vi "PH_Beckhoff.destructor.vi"(0 "i ref in":refnum<vi>, 5 "error in(no error)":errorcluster) -> (19 "error out":errorcluster)   [LabVIEW 2014, in "PH_Beckhoff.lvlib"]
doc: "This is the destructor of a class.\n\nLicense Agreement for this software:\n\nCopyright (C)\nGesellschaft für Schwerionenforschung, GSI\nPlanckstr. 1\n64291 Darmstadt\nGermany\n\nContact: D.Beck@gsi.de \n\nThis program is free software; you can redistribute it and/or modify it under the terms of the \nGNU General Public License as published by the Free Software Foundation; either version 2 of \nthe license, or (at your option) any later version.\n\nThis program is distributed in the hope that it will be useful, but WITHOUT ANY WARRANTY; \nwithout even the implied warranty of MERCHANTABILITY or FITNESS FOR A PARTICULAR PURPOSE. See the GNU General License for more details (http://www.gnu.org).\n\nGesellschaft für Schwerionenforschung, GSI\nPlanckstr. 1, 64291 Darmstadt, Germany\nFor all questions and ideas contact: M.Richter@gsi.de, H.Brand@gsi.de or D.Beck@gsi.de.\nLast update: 16-JUN-2004"
uses:
  PH_Beckhoff.lvlib
  non_GPL/instr.lib/Beckhoff/Beckhoff - Driver np.lvlib
  lib.lib/DimLVEvent/LVDimInterface/LVDimInterface.lvlib
  PH_Class/PH_Class.lvlib
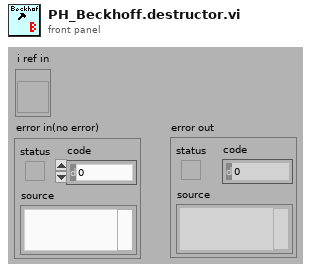
[diagram p1: front panel]
types:
  T1 = typedef "PH_Beckhoff.lvlib/PH_Beckhoff.i attribute.ctl" = cluster{"GUI Refs":T2, "operation?":bool, "Default Prdc Interval":i32, "Connection":T3, "AMS Net ID":T4, "Klemmencluster: # of":T5, "Values":T6, "IP":string, "Description":string, "configured?":bool, "Change Manager":cluster{"Detemination wanted?":bool, "Values changed at":cluster{"Sonderklemmen Inputs":i32[], "Analog Inputs":i32[], "Analog Outputs":i32[], "Digital Inputs":i32[], "Digital Outputs":i32[]}}, "Difference to handle an analog input as change":u32}
  T2 = typedef "PH_Beckhoff.lvlib/PH_Beckhoff.GUI Refs.ctl" = cluster{"ADS Error":refnum<vi>, "Values":refnum<vi>, "configured?":refnum<vi>, "Connection":refnum<vi>, "IP":refnum<vi>, "Prdc Int [ms]":refnum<vi>}
  T3 = typedef "PH_Beckhoff.lvlib/PH_Beckhoff.Connectivity.ctl" = cluster{"DLL?":bool, "Port?":bool, "Client?":bool, "Ping?":bool, "unsuccessful Pings":u32}
  T4 = typedef "Beckhoff - Driver np.lvlib/Beckhoff Access.ctl" = cluster{"DLL path":path, "AMS Net ID":cluster{"1st # of IP":u8, "2nd # of IP":u8, "3rd # of IP":u8, "4th # of IP":u8, "In Port":u8, "Out Port":u8}}
  T5 = typedef "Beckhoff - Driver np.lvlib/Klemmendeclarer.ctl" = cluster{"Offset due to Sonderklemms":u32, "analog Inputs":u32, "analog Outputs":u32, "digital Input Bits":u32, "digital Output Bits":u32}
  T6 = typedef "PH_Beckhoff.lvlib/PH_Beckhoff.Values.ctl" = cluster{"Sonderklemmen Inputs":T7, "Analog Inputs":T8, "Analog Outputs":T10, "Digital Inputs":T11, "Digital Outputs":T12}
  T7 = typedef "PH_Beckhoff.lvlib/PH_Beckhoff.Sonderklemmen Inputs.ctl" = cluster{"Total Length":u32, "Name":string, "Value":u64, "Quality":bool, "Service ID":i32, "Offset":u32, "Length":u32}[]
  T8 = typedef "PH_Beckhoff.lvlib/PH_Beckhoff.Analog Inputs.ctl" = cluster{"Name":string, "Value":u32, "Quality":bool, "Service ID":i32, "Sca Type":T9}[]
  T9 = typedef "PH_Beckhoff.lvlib/PH_Beckhoff.Scaling Type.ctl" = enum16{"none", "0 ... 15 Bit -> 0 ... 5", "0 ... 15 Bit -> 0 ... 10", "0 ... 15 Bit -> 0 ... 25", "0 ... 15 Bit -> 4 ... 20", "0 ... 15 Bit -> 0 ... 1", "0 ... 15 Bit -> 0 ... 20000", "0 ... 15 Bit -> 0 ... 24000"}
  T10 = typedef "PH_Beckhoff.lvlib/PH_Beckhoff.Analog Outputs.ctl" = cluster{"Name":string, "Value":u32, "Quality":bool, "Wanted Value":u32, "Service ID":i32, "Sca Type":T9}[]
  T11 = typedef "PH_Beckhoff.lvlib/PH_Beckhoff.Digital Inputs.ctl" = cluster{"Name":string, "Value":bool, "Quality":bool, "Service ID":i32, "inverted?":bool}[]
  T12 = typedef "PH_Beckhoff.lvlib/PH_Beckhoff.Digital Outputs.ctl" = cluster{"Name":string, "Value":bool, "Quality":bool, "Wanted Value":bool, "Service ID":i32, "inverted?":bool}[]
  T13 = enum16{"SetAttribute", "GetAttribute", "CreateAttribute", "DestroyAttribute", "DestroyAllAtributes"}
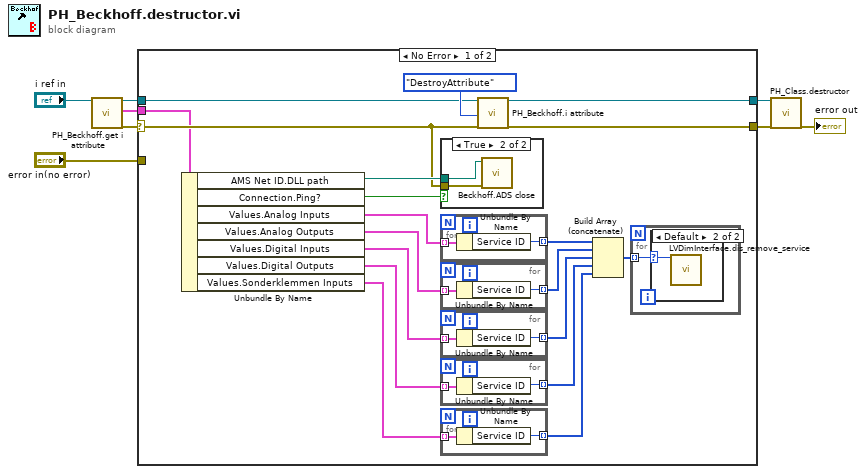
[diagram p0: block diagram]
diagram:
  n1 = call "PH_Beckhoff.get i attribute.vi"("i ref in"="i ref in") -> ("i ref out"=w8:refnum<vi>, "i attribute"=w4:T1, "error out"=w5:errorcluster)  [unwired: 16 in]
  n2 = case shown="No Error" w5 {
    selector: w5 -> [w10 _]
    tunnel: "error in(no error)" -> [_ w42]
    tunnel: w8 -> [w12 w43]
    tunnel: [w13 w42] -> w7
    tunnel: [w11 w43] -> w6
    tunnel: w4 -> [w9 _]
    frame No Error {
      n3 = Unbundle By Name(w9) -> ("AMS Net ID.DLL path"=w14:path, "Connection.Ping?"=w26:bool, "Values.Analog Inputs"=w25:T8, "Values.Analog Outputs"=w24:T10, "Values.Digital Inputs"=w23:T11, "Values.Digital Outputs"=w22:T12, "Values.Sonderklemmen Inputs"=w16:T7)
      n4 = case shown="True" w26 {
        tunnel: w10 -> [_ w41]
        tunnel: w14 -> [_ w40]
        frame False {
        }
        frame True {
          n5 = call "Beckhoff.ADS close.vi"("error in"=w41, "path in"=w40) -> ()  [unwired: 4 in, 2 out]
        }
      }
      n6 = for {
        tunnel: w25 -> [w39] mode=indexing
        tunnel: [w38] -> w21 mode=indexing
        n7 = Unbundle By Name(w39) -> ("Service ID"=w38:i32)
      }
      n8 = for {
        tunnel: w24 -> [w35] mode=indexing
        tunnel: [w34] -> w20 mode=indexing
        n9 = Unbundle By Name(w35) -> ("Service ID"=w34:i32)
      }
      n10 = for {
        tunnel: w23 -> [w33] mode=indexing
        tunnel: [w32] -> w19 mode=indexing
        n11 = Unbundle By Name(w33) -> ("Service ID"=w32:i32)
      }
      n12 = for {
        tunnel: w22 -> [w31] mode=indexing
        tunnel: [w30] -> w18 mode=indexing
        n13 = Unbundle By Name(w31) -> ("Service ID"=w30:i32)
      }
      n14 = for {
        tunnel: w16 -> [w29] mode=indexing
        tunnel: [w28] -> w15 mode=indexing
        n15 = Unbundle By Name(w29) -> ("Service ID"=w28:i32)
      }
      n16 = call "PH_Beckhoff.i attribute.vi"("VI Refnum"=w12, "Action"=T13."DestroyAttribute", "error in (no error)"=w10) -> ("VI Refnum out"=w11:refnum<vi>, "error out"=w13:errorcluster)  [unwired: 14 in, 1 out]
      n17 = Build Array (concatenate)(w21, w20, w19, w18, w15) -> (w17:i32[])
      n18 = for {
        tunnel: w17 -> [w36] mode=indexing
        n19 = case shown="Default" w36 {
          selector: w36 -> [_ w37]
          frame -1 {
          }
          frame Default {
            n20 = call "LVDimInterface.dis_remove_service.vi"("my_serviceID"=w37) -> ()  [unwired: 18 in, 1 out]
          }
        }
      }
    }
    frame Error {
    }
  }
  n21 = call "PH_Class.destructor.vi"("i ref in"=w6, "error in(no error)"=w7) -> ("error out"=→"error out":errorcluster)  [unwired: 17 in]
